vi "California Instruments iX Series Waveform Display.vi"() -> ()   [LabVIEW 2011]
doc: "Demonstrates acquiring multiple Voltage or Current measurement and displaying it in waveform."
uses:
  <instrlib>/California Instruments iX Series/Public/Data/Read Multiple Voltage Measurements.vi
  <instrlib>/California Instruments iX Series/Public/Data/Read Multiple Current Measurements.vi
  <instrlib>/California Instruments iX Series/California Instruments iX Series.lvlib
panel:
  in  "Serial Configuration":cluster{"Baud Rate":u32, "Flow Control":u16}={"Baud Rate"=460800, "Flow Control"=0} {"Flow Control" items=["None", "XON/XOFF", "RTS/CTS", "XON/XOFF & RTS/CTS", "DTR/DSR", "XON/XOFF & DTR/DSR"]; "Baud Rate" items=["9600"=9600, "19200"=19200, "38400"=38400, "57600"=57600, "115200"=115200, "230400"=230400, "460800"=460800]}
  out "Waveform Graph":sgl[](graph)
  in  "VISA resource name":refnum<visa-resource-name>
  in  "Stop":bool
  in  "Active Phase (1:Phase 1)":i32(ring)=1 items=["Phase 1"=1, "Phase 2"=2, "Phase 3"=3]
  in  "Voltage/Current (0:Voltage)":u16(ring) items=["Voltage", "Current"]
  # "(c) 2009 National Instruments.  ALL RIGHTS RESERVED."
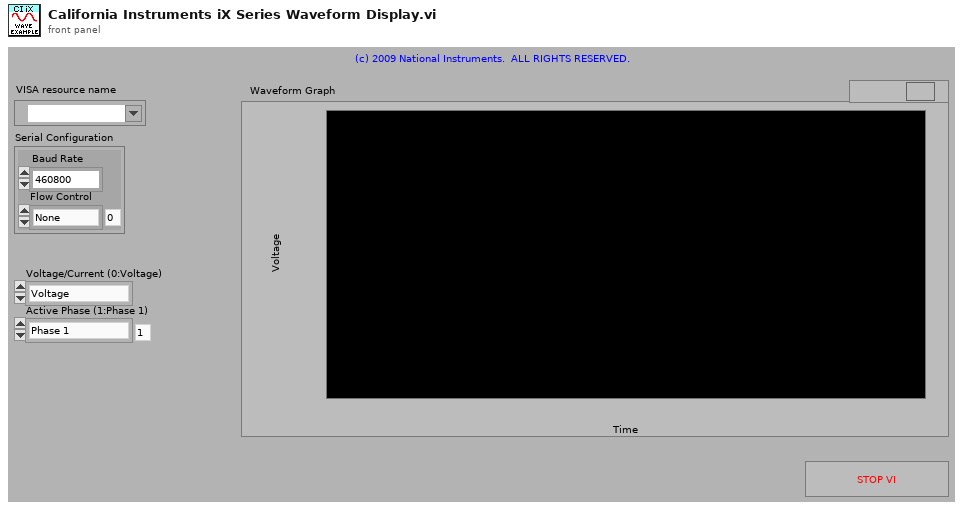
[diagram p1: front panel]
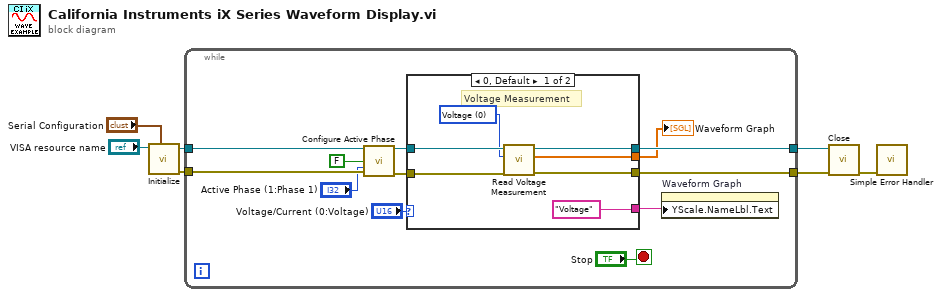
[diagram p0: block diagram]
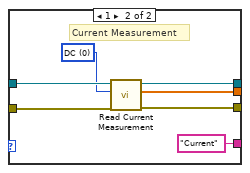
[diagram p2: hidden frame]
diagram:
  n1 = call <instrlib>:"Initialize.vi"("Serial Configuration"="Serial Configuration", "VISA resource name"="VISA resource name") -> ("error out"=w6:errorcluster, "VISA resource name out"=w7:refnum<visa-resource-name>)  [unwired: 8 in]
  n2 = while {
    tunnel: w7 -> [w16]
    tunnel: w6 -> [w15]
    tunnel: [w10] -> w2
    tunnel: [w9] -> w3
    stop <- "Stop" stop-if-true
    n3 = call <instrlib>:"Configure Active Phase.vi"("VISA resource name"=w16, "Enable Coupling (Enabled)"=FALSE ("Enabled Coupling (Enabled)"), "Active Phase (1:Phase 1)"="Active Phase (1:Phase 1)", "error in (no error)"=w15) -> ("VISA resource name out"=w18:refnum<visa-resource-name>, "error out"=w17:errorcluster)  [unwired: 10 in]
    n4 = case shown="0, Default" "Voltage/Current (0:Voltage)" {
      tunnel: w18 -> [w26 w33]
      tunnel: w17 -> [w25 w32]
      tunnel: [w22 w31] -> w8
      tunnel: [w24 w30] -> w10
      tunnel: [w23 w29] -> w9
      tunnel: ["Voltage" "Current"] -> w11
      frame 0, Default {
        w21 = u16 0 items=["Voltage", "Voltage Harmonic Amplitude", "Voltage Harmonic Phase"] ("Multiple Voltage Measurement Type (0:DC)")
        # "Voltage Measurement"
        n5 = call-poly <instrlib>:"Read Voltage Measurement.vi"("error in (no error)"=w25, "Multiple Voltage Measurement Type (0:DC)"=w21, "VISA resource name"=w26) -> ("error out"=w23:errorcluster, "Voltage Measurements"=w22:sgl[], "VISA resource name out"=w24:refnum<visa-resource-name>)  [unwired: 6 in]
      }
      frame 1 {
        w28 = u16 0 items=["DC", "Current Harmonic Amplitude", "Current Harmonic Phase", "Neutral DC Current", "Neutral Current Harmonic Amplitude", "Neutral Current Harmonic Phase"] ("Multiple Current Measurement Type (0:DC)")
        # "Current Measurement"
        n6 = call-poly <instrlib>:"Read Current Measurement.vi"("error in (no error)"=w32, "Multiple Current Measurement Type (0:DC)"=w28, "VISA resource name"=w33) -> ("error out"=w29:errorcluster, "Current Measurements"=w31:sgl[], "VISA resource name out"=w30:refnum<visa-resource-name>)  [unwired: 6 in]
      }
    }
    "Waveform Graph" <- w8
    n7 = property on="Waveform Graph" class="WFGraph (strict)"("YScale.NameLbl.Text"=w11) -> ()  [unwired: 2 in, 2 out]
  }
  n8 = call <instrlib>:"Close.vi"("error in (no error)"=w3, "VISA resource name"=w2) -> ("error out"=w1:errorcluster)  [unwired: 9 in]
  n9 = call <vilib>:"Simple Error Handler.vi"("error in (no error)"=w1) -> ()  [unwired: 4 in, 5 out]
